vi "Measurement duplicator.vi"(0 "Index in":T1={"IV"=[{"Name"="Test", "Comment"="", "Time"=timestamp(0 s since 1904-01-01), "Folder"=path "", "IV properties"={"T"=0.0, "Vstart"=0.0, "Vstop"=0.0, "Vpoints"=0.0, "Settling"=0.01, "I limit"=0.1, "Log mapping"=FALSE, "Averaging"=0.0}, "GUID"=""}], "CV"=[], "LDLTS"=[], "Conv DLTS"=[]} {"IV"."IV properties"."Settling" min=0.0 max=65535.0; "CV"."CV properties"."V range" items=["10mV"=0.01, "100mV"=0.1, "1V"=1.0, "10V"=10.0]; "CV"."CV properties"."I range" items=["100nA"=-7.0, "1µA"=-6.0, "10µA"=-5.0, "100µA"=-4.0, "1mA"=-3.0, "10mA"=-2.0]; "LDLTS"."LDLTS properties"."V range" items=["10mV"=0.01, "100mV"=0.1, "1V"=1.0, "10V"=10.0]; "LDLTS"."LDLTS properties"."I range" items=["100nA"=-7.0, "1µA"=-6.0, "10µA"=-5.0, "100µA"=-4.0, "1mA"=-3.0, "10mA"=-2.0]; "Conv DLTS"."DLTS properties"."V range" items=["10mV"=0.01, "100mV"=0.1, "1V"=1.0, "10V"=10.0]; "Conv DLTS"."DLTS properties"."I range" items=["10mV"=0.01, "100mV"=0.1, "1V"=1.0, "10V"=10.0]}, 5 "Workspace":path, 7 "Tree tag":string, 11 "error in (no error)":errorcluster) -> (4 "Index out":T1={"IV"=[{"Name"="Test", "Comment"="", "Time"=timestamp(0 s since 1904-01-01), "Folder"=path "", "IV properties"={"T"=0.0, "Vstart"=0.0, "Vstop"=0.0, "Vpoints"=0.0, "Settling"=0.01, "I limit"=0.1, "Log mapping"=FALSE, "Averaging"=0.0}, "GUID"=""}], "CV"=[], "LDLTS"=[], "Conv DLTS"=[]} {"IV"."IV properties"."Settling" min=0.0 max=65535.0; "CV"."CV properties"."V range" items=["10mV"=0.01, "100mV"=0.1, "1V"=1.0, "10V"=10.0]; "CV"."CV properties"."I range" items=["100nA"=-7.0, "1µA"=-6.0, "10µA"=-5.0, "100µA"=-4.0, "1mA"=-3.0, "10mA"=-2.0]; "LDLTS"."LDLTS properties"."V range" items=["10mV"=0.01, "100mV"=0.1, "1V"=1.0, "10V"=10.0]; "LDLTS"."LDLTS properties"."I range" items=["100nA"=-7.0, "1µA"=-6.0, "10µA"=-5.0, "100µA"=-4.0, "1mA"=-3.0, "10mA"=-2.0]; "Conv DLTS"."DLTS properties"."V range" items=["10mV"=0.01, "100mV"=0.1, "1V"=1.0, "10V"=10.0]; "Conv DLTS"."DLTS properties"."I range" items=["10mV"=0.01, "100mV"=0.1, "1V"=1.0, "10V"=10.0]}, 6 "ID":i32, 8 "Type":enum16{"I-V", "C-V", "cDLTS", "LDLTS"}(ring), 10 "Canceled":bool, 15 "error out":errorcluster)   [LabVIEW 2019]
doc: "Handles creation of a new measurement with parameters duplicated from an existing one, displays a GUI window"
uses:
  Type defs/Session internal index Type Def.ctl
  Type defs/IV measurement Type Def.ctl
  Type defs/IV properties Type Def.ctl
  Type defs/CV measurement Type Def.ctl
  Type defs/CV properties Type Def.ctl
  Type defs/LDLTS measurement Type Def.ctl
  Type defs/LDLTS properties Type Def.ctl
  Type defs/cDLTS measurement Type Def.ctl
  Type defs/DLTS properties Type Def.ctl
  <vilib>/Utility/miscctls.llb/LVPointTypeDef.ctl
panel:
  out "Header":string
  in  "Cancel":bool
  in  "Apply":bool
  in  "Comment":string
  in  "Measurment name":string
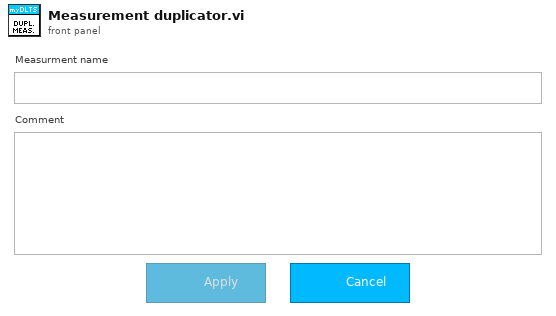
[diagram p1: front panel]
types:
  T1 = typedef "Session internal index Type Def.ctl" = cluster{"IV":T2[], "CV":T4[], "LDLTS":T6[], "Conv DLTS":T8[]}
  T2 = typedef "IV measurement Type Def.ctl" = cluster{"Name":string, "Comment":string, "Time":timestamp, "Folder":path, "IV properties":T3, "GUID":string}
  T3 = typedef "IV properties Type Def.ctl" = cluster{"T":dbl[unit], "Vstart":dbl[unit], "Vstop":dbl[unit], "Vpoints":dbl, "Settling":dbl[unit], "I limit":dbl[unit], "Log mapping":bool, "Averaging":dbl}
  T4 = typedef "CV measurement Type Def.ctl" = cluster{"Name":string, "Comment":string, "Time":timestamp, "Folder":path, "CV properties":T5, "GUID":string}
  T5 = typedef "CV properties Type Def.ctl" = cluster{"T":dbl[unit], "Vstart":dbl[unit], "Vstop":dbl[unit], "Vpoints":dbl, "Precision":enum16{"Low (Fast)", "Normal", "High (Slow)"}, "Test signal":dbl[unit], "Auto I range":bool, "Test frequency":dbl[unit], "I range":dbl, "V range":dbl[unit], "Log mapping":bool, "Rel perm":dbl, "Area":dbl[unit]}
  T6 = typedef "LDLTS measurement Type Def.ctl" = cluster{"Name":string, "Comment":string, "Time":timestamp, "Folder":path, "LDLTS properties":T7, "GUID":string}
  T7 = typedef "LDLTS properties Type Def.ctl" = cluster{"T":dbl[unit], "Test signal":dbl[unit], "Test frequency":dbl[unit], "Bandwidth":dbl[unit], "Averaging":dbl, "Vbias":dbl[unit], "Vpulse":dbl[unit], "pulse length":dbl[unit], "Pulse 2":bool, "Vpulse 2":dbl[unit], "pulse length 2":dbl[unit], "I range":dbl, "V range":dbl[unit], "Sampling rate":dbl[unit], "Acq. delay":dbl[unit], "Sampling time":dbl[unit]}
  T8 = typedef "cDLTS measurement Type Def.ctl" = cluster{"Name":string, "Comment":string, "Time":timestamp, "Folder":path, "DLTS properties":T9, "GUID":string}
  T9 = typedef "DLTS properties Type Def.ctl" = cluster{"Tstart":dbl[unit], "Instant start":bool, "Tstop":dbl[unit], "T rate":dbl[unit], "Test signal":dbl[unit], "Test frequency":dbl[unit], "Bandwidth":dbl[unit], "Averaging":dbl, "Vbias":dbl[unit], "Vpulse":dbl[unit], "pulse length":dbl[unit], "Pulse 2":bool, "Vpulse 2":dbl[unit], "pulse length 2":dbl[unit], "I range":dbl, "V range":dbl[unit], "Emission rate":dbl[unit][], "Sampling rate":dbl[unit], "Acq. delay":dbl[unit]}
  T10 = enum8{"Enabled", "Disabled", "Disabled and Grayed Out"}
  T11 = typedef "LVPointTypeDef.ctl" = cluster{"Horizontal":i16, "Vertical":i16}
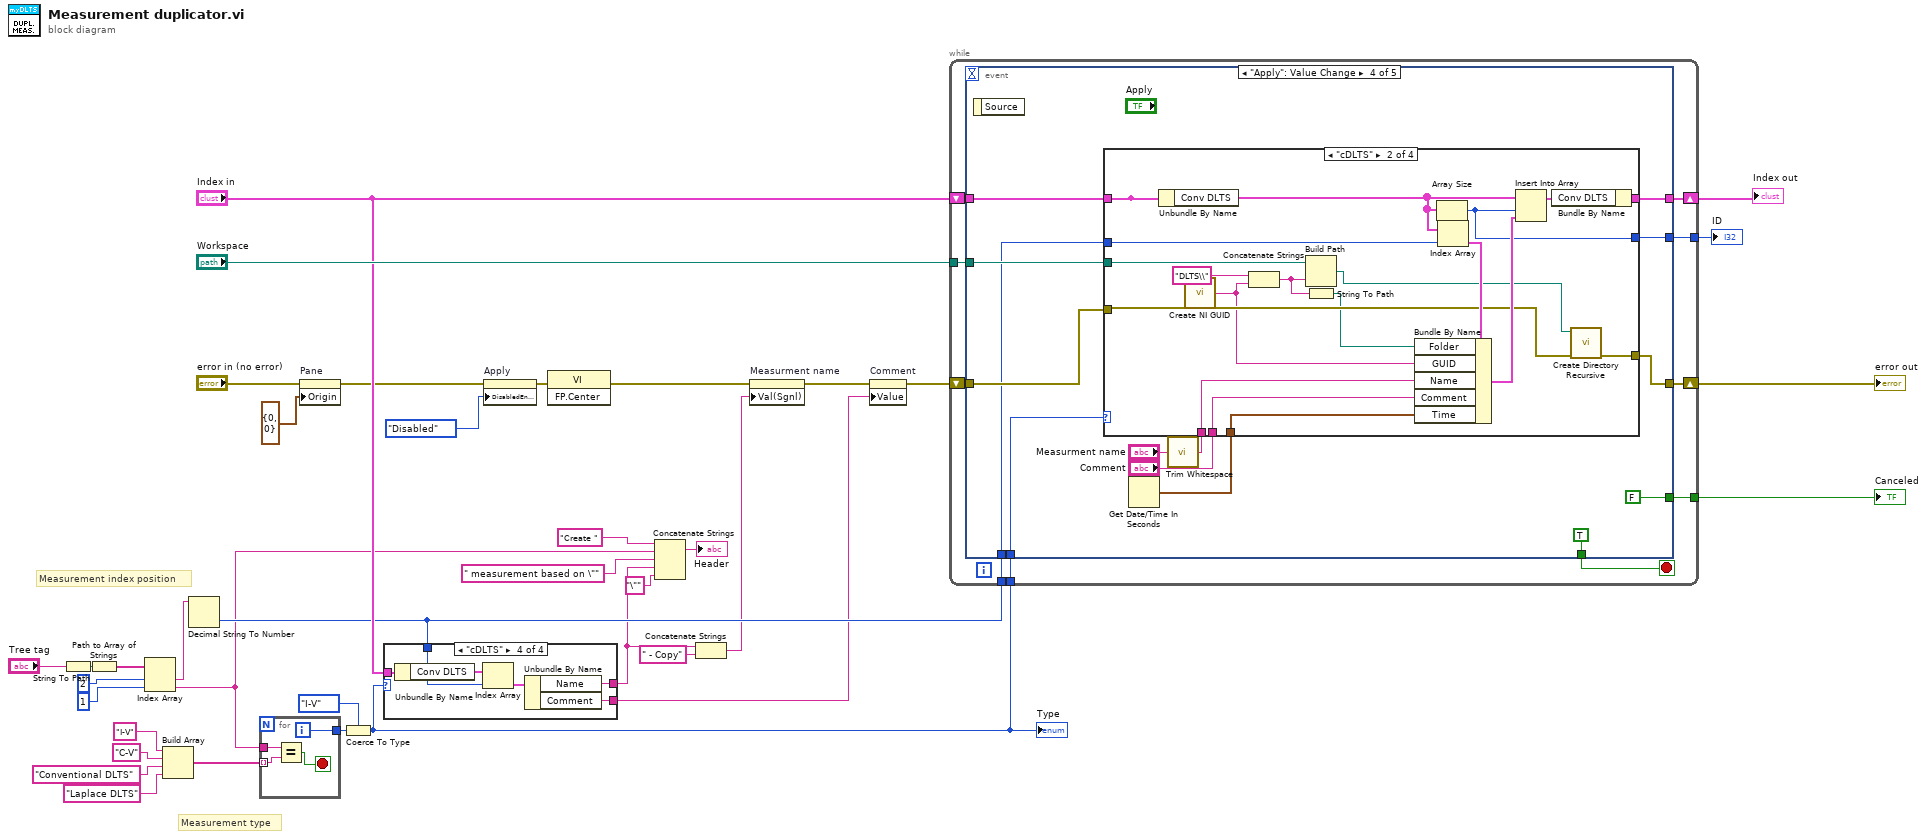
[diagram p0: block diagram]
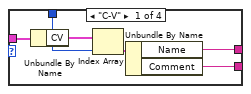
[diagram p2: hidden frame]
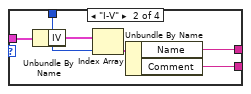
[diagram p3: hidden frame]
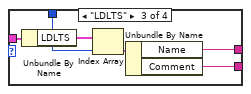
[diagram p4: hidden frame]
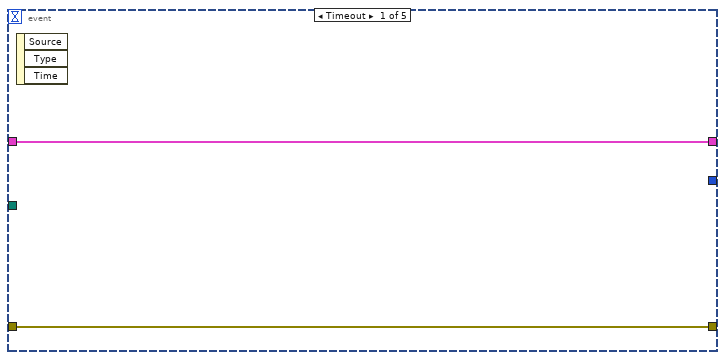
[diagram p5: hidden frame]
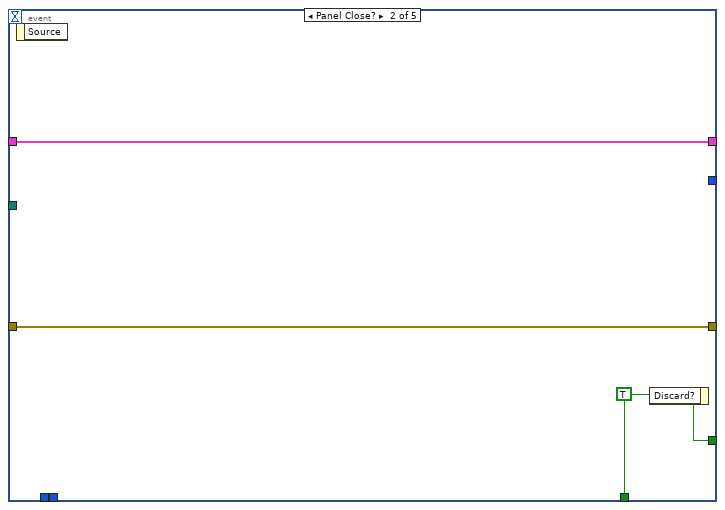
[diagram p6: hidden frame]
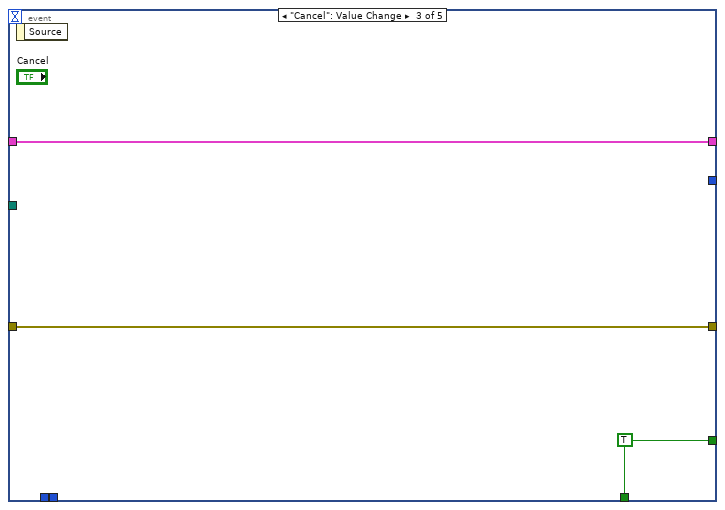
[diagram p7: hidden frame]
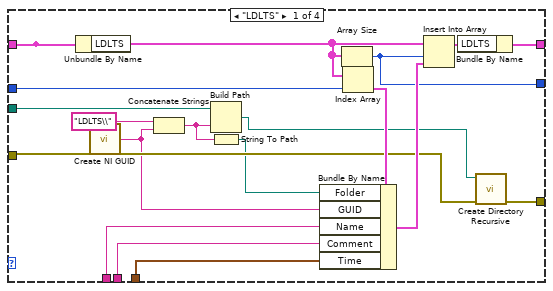
[diagram p8: hidden frame]
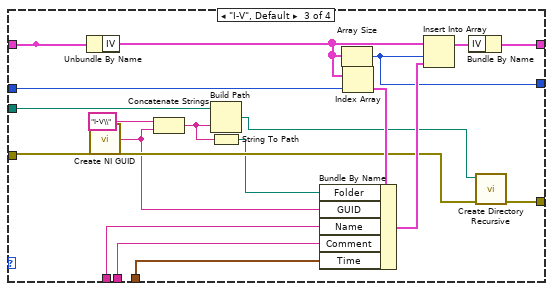
[diagram p9: hidden frame]
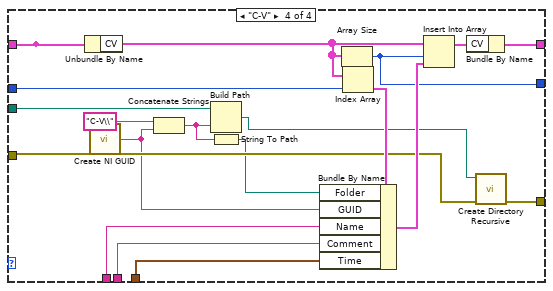
[diagram p10: hidden frame]
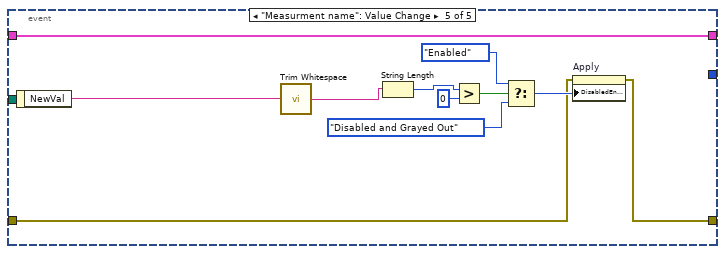
[diagram p11: hidden frame]
diagram:
  # "Measurement type"
  # "Measurement index position"
  n1 = String To Path(string="Tree tag") -> (path=w27:path)
  n2 = Path to Array of Strings(0:w27) -> (2:w28:string[])  [unwired: 1 out]
  n3 = Index Array(array=w28, index #1=2 ("index"), index #2=1 ("index")) -> (element #1=w29:string, element #2=w11:string)
  n4 = Build Array("I-V", "C-V" ("element"), "Conventional DLTS" ("element"), "Laplace DLTS" ("element")) -> (w25:string[])
  n5 = Decimal String To Number(string=w29) -> (number=w14:i32)  [unwired: 2 in, 1 out]
  n6 = for {
    tunnel: w25 -> [w42] mode=indexing
    tunnel: [w41] -> w26
    tunnel: w11 -> [w39]
    i -> [w41]
    stop <- w40 stop-if-true
    n7 = Equal?(x=w39, y=w42) -> (x = y?=w40:bool)
  }
  n8 = property on="Pane" class="Pane"(error in="error in (no error)", "Origin"=T11 {"Horizontal"=0, "Vertical"=0}) -> (error out=w6:errorcluster)  [unwired: 1 in, 1 out]
  n9 = Coerce To Type(0:w26, 1:enum16{"I-V", "C-V", "cDLTS", "LDLTS"}."I-V") -> (2:w16:enum16{"I-V", "C-V", "cDLTS", "LDLTS"})
  "Type" <- w16
  n10 = case shown="\"cDLTS\"" w16 {
    tunnel: "Index in" -> [w48 w54 w60 w66]
    tunnel: w14 -> [w46 w52 w58 w64]
    tunnel: [w44 w50 w56 w62] -> w8
    tunnel: [w43 w49 w55 w61] -> w4
    frame "C-V" {
      n11 = Unbundle By Name(w48) -> ("CV"=w47:T4[])
      n12 = Index Array(array=w47, index=w46) -> (element=w45:T4)
      n13 = Unbundle By Name(w45) -> ("Name"=w44:string, "Comment"=w43:string)
    }
    frame "I-V" {
      n14 = Unbundle By Name(w54) -> ("IV"=w53:T2[])
      n15 = Index Array(array=w53, index=w52) -> (element=w51:T2)
      n16 = Unbundle By Name(w51) -> ("Name"=w50:string, "Comment"=w49:string)
    }
    frame "LDLTS" {
      n17 = Unbundle By Name(w60) -> ("LDLTS"=w59:T6[])
      n18 = Index Array(array=w59, index=w58) -> (element=w57:T6)
      n19 = Unbundle By Name(w57) -> ("Name"=w56:string, "Comment"=w55:string)
    }
    frame "cDLTS" {
      n20 = Unbundle By Name(w66) -> ("Conv DLTS"=w65:T8[])
      n21 = Index Array(array=w65, index=w64) -> (element=w63:T8)
      n22 = Unbundle By Name(w63) -> ("Name"=w62:string, "Comment"=w61:string)
    }
  }
  n23 = property on="Apply" class="Bool"(error in=w6, "DisabledEnum"=T10."Disabled" ("Disabled")) -> (error out=w30:errorcluster)  [unwired: 1 in, 1 out]
  n24 = invoke class="VI" method="FP.Center"(error in=w30) -> (error out=w3:errorcluster)  [unwired: 2 in, 2 out]
  n25 = Concatenate Strings("Create " ("string"), w11, " measurement based on \"" ("string"), w8, "\"" ("string")) -> (→"Header":string)
  n26 = Concatenate Strings(w8, " - Copy" ("string")) -> (w5:string)
  n27 = property on="Measurment name" class="Str"(error in=w3, "Val(Sgnl)"=w5) -> (error out=w1:errorcluster)  [unwired: 1 in, 1 out]
  n28 = property on="Comment" class="Str"(error in=w1, "Value"=w4) -> (error out=w2:errorcluster)  [unwired: 1 in, 1 out]
  n29 = while {
    tunnel: [w75] -> w38
    shift-right: [w73] -> w36
    shift-left: w2 -> [w74]
    tunnel: "Workspace" -> [w71]
    tunnel: [w69] -> w31
    shift-right: [w70] -> w32
    shift-left: "Index in" -> [w72]
    tunnel: w16 -> [w68]
    tunnel: w14 -> [w67]
    stop <- w76 stop-if-true
    n30 = event shown="[3] \"Apply\": Value Change" {
      selector: _ -> [_ _ _ _ _]
      dyn-events: _ -> [_ _ _ _ _]
      timeout: _ -> [_ _ _ _ _]
      tunnel: [_ w81 w84 TRUE ("Discard?") _] -> w76
      tunnel: [_ w81 w84 FALSE ("Discard?") _] -> w75
      tunnel: w74 -> [w78 w80 w83 w87 w180]
      tunnel: [w78 w80 w83 w89 w181] -> w73
      tunnel: w72 -> [w77 w79 w82 w95 w175]
      tunnel: w71 -> [_ _ _ w91 _]
      tunnel: [w77 w79 w82 w90 w175] -> w70
      tunnel: [_ _ _ w88 _] -> w69
      tunnel: w68 -> [_ _ _ w86 _]
      tunnel: w67 -> [_ _ _ w85 _]
      event Timeout {
        n31 = event-data() -> ()  [unwired: 1 in, 3 out]
      }
      event Panel Close? {
        w81 = TRUE ("Discard?")
        n32 = event-data() -> ()  [unwired: 1 in, 1 out]
        n33 = event-data("Discard?"=w81) -> ()  [unwired: 1 in, 1 out]
      }
      event "Cancel": Value Change {
        w84 = TRUE ("Discard?")
        n34 = event-data() -> ()  [unwired: 1 in, 1 out]
      }
      event "Apply": Value Change {
        n35 = event-data() -> ()  [unwired: 1 in, 1 out]
        n36 = Get Date/Time In Seconds() -> (seconds since 1Jan1904=w92:timestamp)
        n37 = call <vilib>:"Trim Whitespace.vi"("string"="Measurment name") -> ("trimmed string"=w94:string)  [unwired: 1 in]
        n38 = case shown="\"cDLTS\"" w86 {
          tunnel: w95 -> [w110 w129 w148 w167]
          tunnel: w94 -> [w117 w136 w155 w174]
          tunnel: "Comment" -> [w116 w135 w154 w173]
          tunnel: w92 -> [w114 w133 w152 w171]
          tunnel: w91 -> [w102 w121 w140 w159]
          tunnel: [w109 w128 w147 w166] -> w90
          tunnel: [w111 w130 w149 w168] -> w89
          tunnel: [w107 w126 w145 w164] -> w88
          tunnel: w87 -> [w103 w122 w141 w160]
          tunnel: w85 -> [w106 w125 w144 w163]
          frame "LDLTS" {
            n39 = Unbundle By Name(w110) -> ("LDLTS"=w112:T6[])
            n40 = call "Create NI GUID.vi"() -> ("NI GUID"=w99:string)
            n41 = Concatenate Strings("LDLTS\\" ("string"), w99) -> (w105:string)
            n42 = Build Path(base path=w102, name or relative path=w105) -> (appended path=w101:path)
            n43 = String To Path(string=w105) -> (path=w100:path)
            n44 = Array Size(array=w112) -> (size(s)=w107:i32)
            n45 = Index Array(array=w112, index=w106) -> (element=w115:T6)
            n46 = Bundle By Name(cluster=w115, "Folder"=w100, "GUID"=w99, "Name"=w117, "Comment"=w116, "Time"=w114) -> (w113:T6)
            n47 = Insert Into Array(array=w112, index=w107, new element=w113) -> (w108:T6[])
            n48 = Bundle By Name(cluster=w110, "LDLTS"=w108) -> (w109:T1)
            n49 = call <vilib>:"Create Directory Recursive.vi"("error in (no error)"=w103, "directory"=w101) -> ("error out"=w111:errorcluster)  [unwired: 3 in, 2 out]
          }
          frame "cDLTS" {
            n50 = Unbundle By Name(w129) -> ("Conv DLTS"=w131:T8[])
            n51 = call "Create NI GUID.vi"() -> ("NI GUID"=w118:string)
            n52 = Concatenate Strings("DLTS\\" ("string"), w118) -> (w124:string)
            n53 = Build Path(base path=w121, name or relative path=w124) -> (appended path=w120:path)
            n54 = String To Path(string=w124) -> (path=w119:path)
            n55 = Array Size(array=w131) -> (size(s)=w126:i32)
            n56 = Index Array(array=w131, index=w125) -> (element=w134:T8)
            n57 = Bundle By Name(cluster=w134, "Folder"=w119, "GUID"=w118, "Name"=w136, "Comment"=w135, "Time"=w133) -> (w132:T8)
            n58 = Insert Into Array(array=w131, index=w126, new element=w132) -> (w127:T8[])
            n59 = Bundle By Name(cluster=w129, "Conv DLTS"=w127) -> (w128:T1)
            n60 = call <vilib>:"Create Directory Recursive.vi"("error in (no error)"=w122, "directory"=w120) -> ("error out"=w130:errorcluster)  [unwired: 3 in, 2 out]
          }
          frame "I-V", Default {
            n61 = Unbundle By Name(w148) -> ("IV"=w150:T2[])
            n62 = call "Create NI GUID.vi"() -> ("NI GUID"=w137:string)
            n63 = Concatenate Strings("I-V\\" ("string"), w137) -> (w143:string)
            n64 = Build Path(base path=w140, name or relative path=w143) -> (appended path=w139:path)
            n65 = String To Path(string=w143) -> (path=w138:path)
            n66 = Array Size(array=w150) -> (size(s)=w145:i32)
            n67 = Index Array(array=w150, index=w144) -> (element=w153:T2)
            n68 = Bundle By Name(cluster=w153, "Folder"=w138, "GUID"=w137, "Name"=w155, "Comment"=w154, "Time"=w152) -> (w151:T2)
            n69 = Insert Into Array(array=w150, index=w145, new element=w151) -> (w146:T2[])
            n70 = Bundle By Name(cluster=w148, "IV"=w146) -> (w147:T1)
            n71 = call <vilib>:"Create Directory Recursive.vi"("error in (no error)"=w141, "directory"=w139) -> ("error out"=w149:errorcluster)  [unwired: 3 in, 2 out]
          }
          frame "C-V" {
            n72 = Unbundle By Name(w167) -> ("CV"=w169:T4[])
            n73 = call "Create NI GUID.vi"() -> ("NI GUID"=w156:string)
            n74 = Concatenate Strings("C-V\\" ("string"), w156) -> (w162:string)
            n75 = Build Path(base path=w159, name or relative path=w162) -> (appended path=w158:path)
            n76 = String To Path(string=w162) -> (path=w157:path)
            n77 = Array Size(array=w169) -> (size(s)=w164:i32)
            n78 = Index Array(array=w169, index=w163) -> (element=w172:T4)
            n79 = Bundle By Name(cluster=w172, "Folder"=w157, "GUID"=w156, "Name"=w174, "Comment"=w173, "Time"=w171) -> (w170:T4)
            n80 = Insert Into Array(array=w169, index=w164, new element=w170) -> (w165:T4[])
            n81 = Bundle By Name(cluster=w167, "CV"=w165) -> (w166:T1)
            n82 = call <vilib>:"Create Directory Recursive.vi"("error in (no error)"=w160, "directory"=w158) -> ("error out"=w168:errorcluster)  [unwired: 3 in, 2 out]
          }
        }
      }
      event "Measurment name": Value Change {
        n83 = event-data() -> ("NewVal"=w183:string)  [unwired: 1 in]
        n84 = call <vilib>:"Trim Whitespace.vi"("string"=w183) -> ("trimmed string"=w179:string)  [unwired: 1 in]
        n85 = String Length(string=w179) -> (length=w177:i32)
        n86 = Greater?(x=w177, y=0) -> (0:w176:bool)
        n87 = Select(t=T10."Enabled" ("Disabled"), s=w176, f=T10."Disabled and Grayed Out") -> (s? t:f=w182:T10)
        n88 = property on="Apply" class="Bool"(error in=w180, "DisabledEnum"=w182) -> (error out=w181:errorcluster)  [unwired: 1 in, 1 out]
      }
    }
  }
  "Canceled" <- w38
  "error out" <- w36
  "Index out" <- w32
  "ID" <- w31
